vi "Formate into SQL Report.vi"(8 "error in (no error)":errorcluster) -> (0 "error out":errorcluster, 3 "Result for SQl Without Header":string[][](array[string]))   [LabVIEW 2017]
uses:
  <vilib>/Utility/file.llb/Read Delimited Spreadsheet (string).vi
panel:
  in  "file path (dialog if empty)":path=path "D:/STD EOL/MSSQL Report Viewer/IOT/Report/Sample Reports/Report/Test Report/Main Reports/21-05-19.csv"
  in  "Excepted Value":string="Excepted Value"
  in  "Test Type":string="Test type"
  out "Result wiht Header":string[][](array[string])
  in  "Variant":string="variant"
  in  "Model":string="Y1k"
  in  "Shift":string="A"
  in  "User Name":string="mmk"
  in  "Barcode":string="123"
  out "all rows":string[][](array[string])
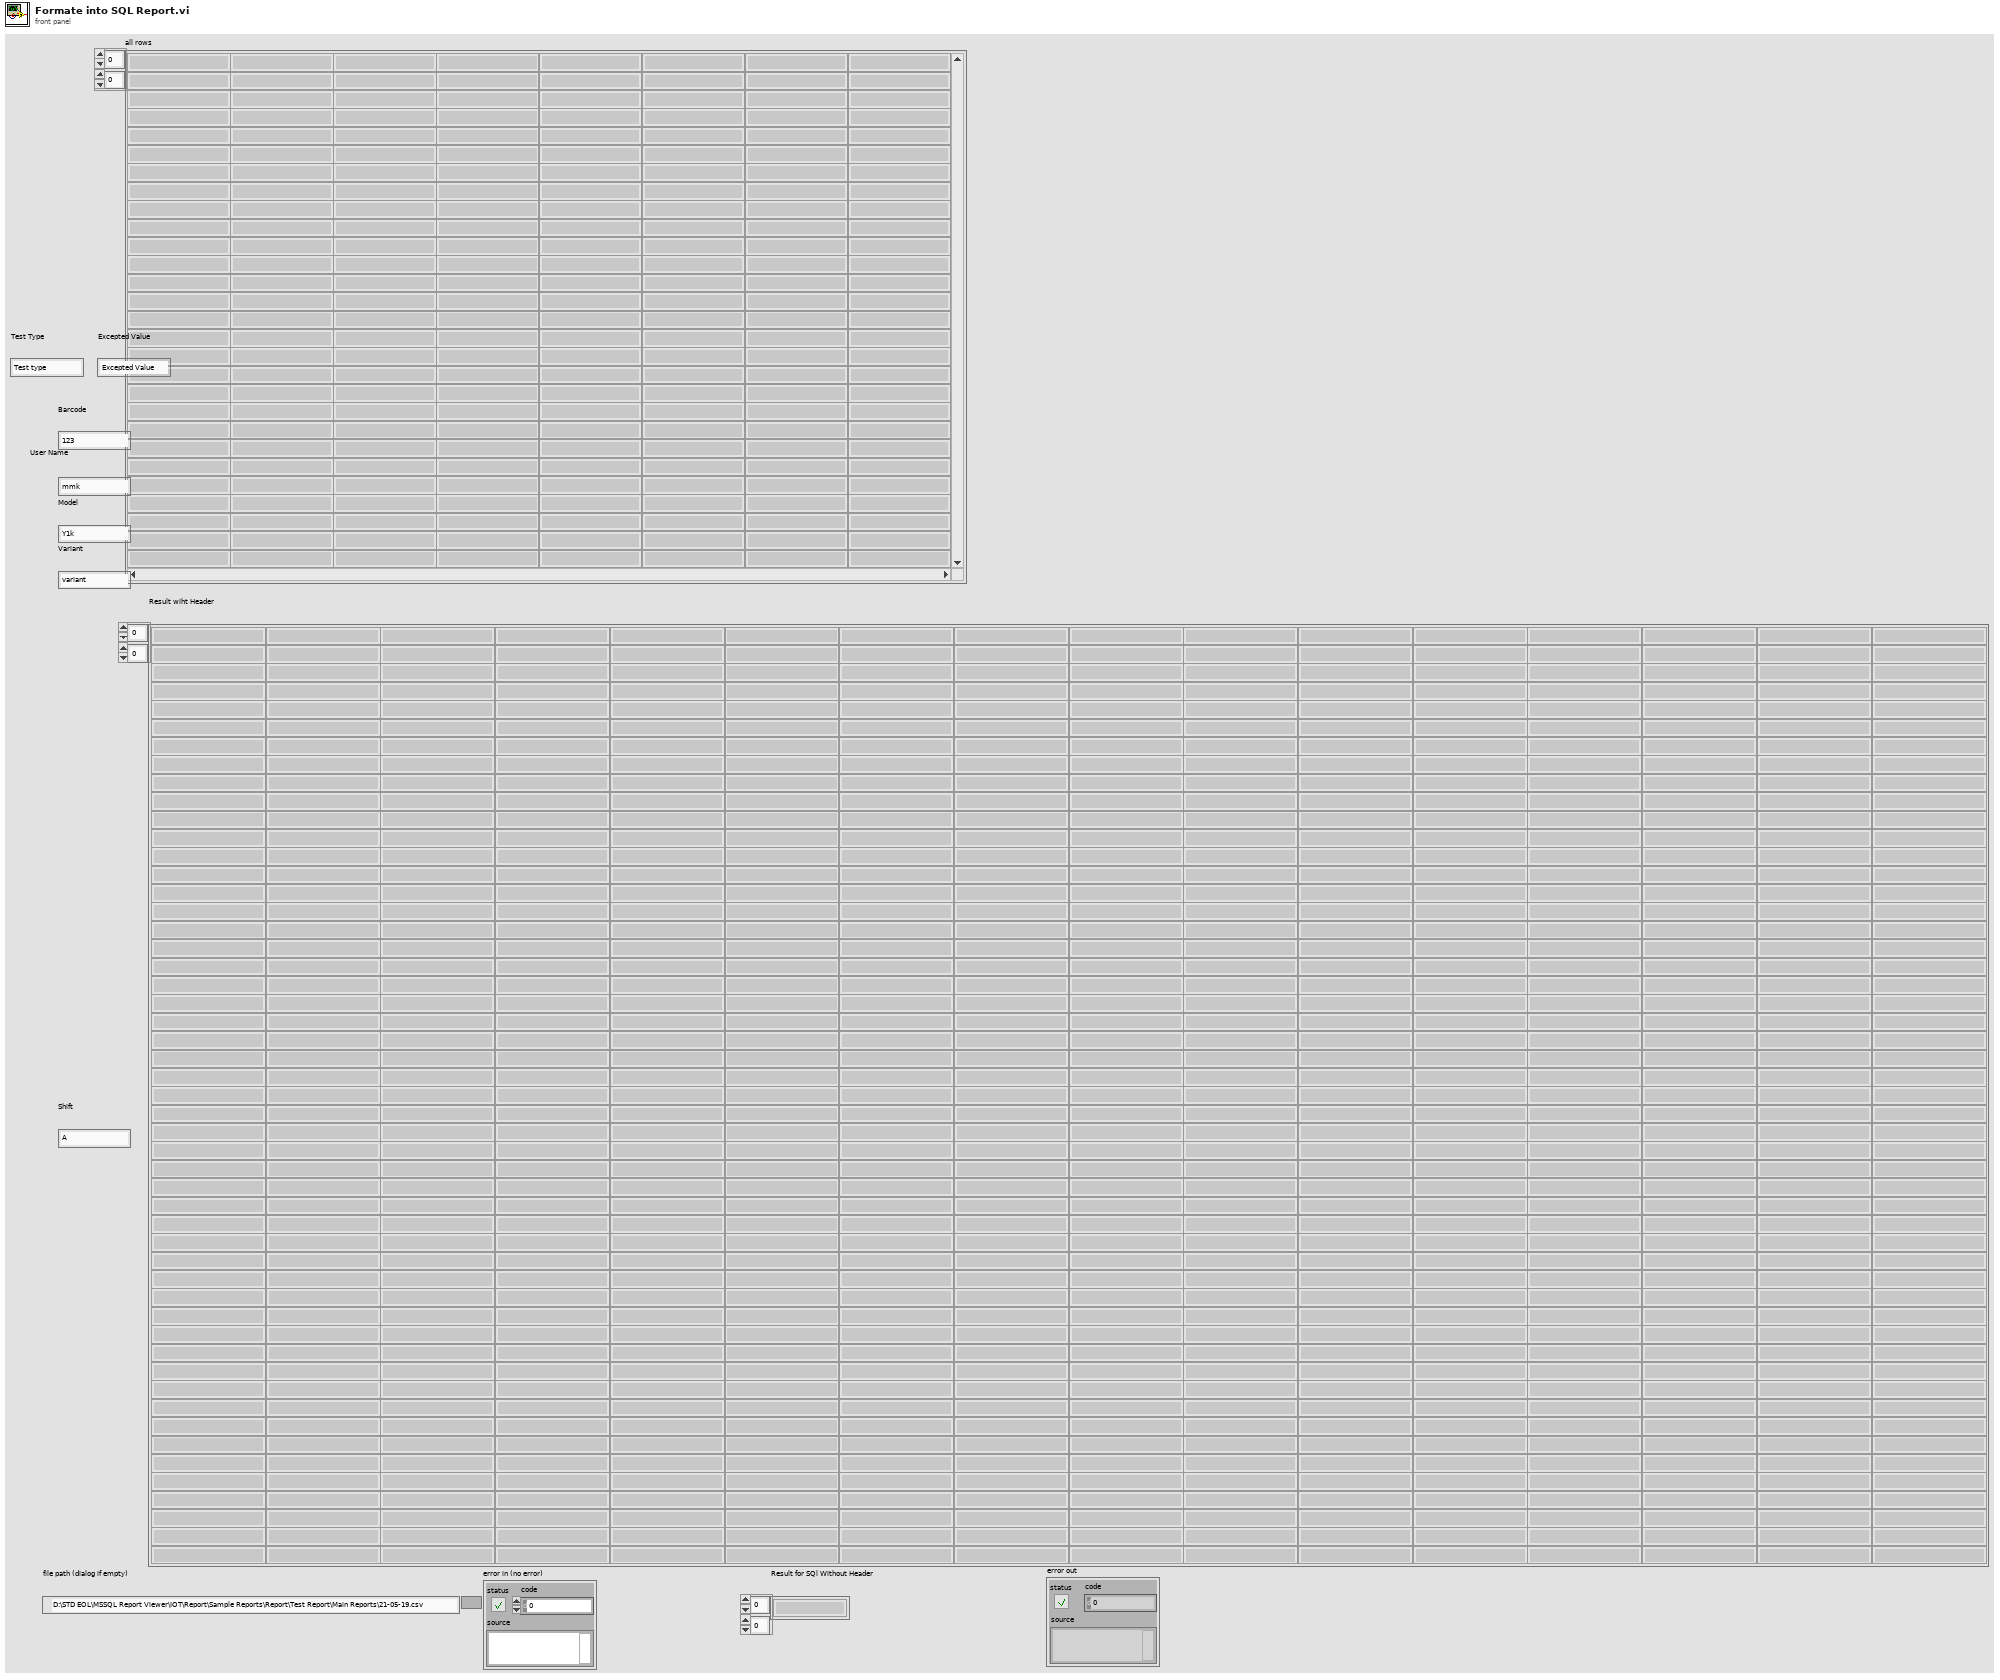
[diagram p1: front panel]
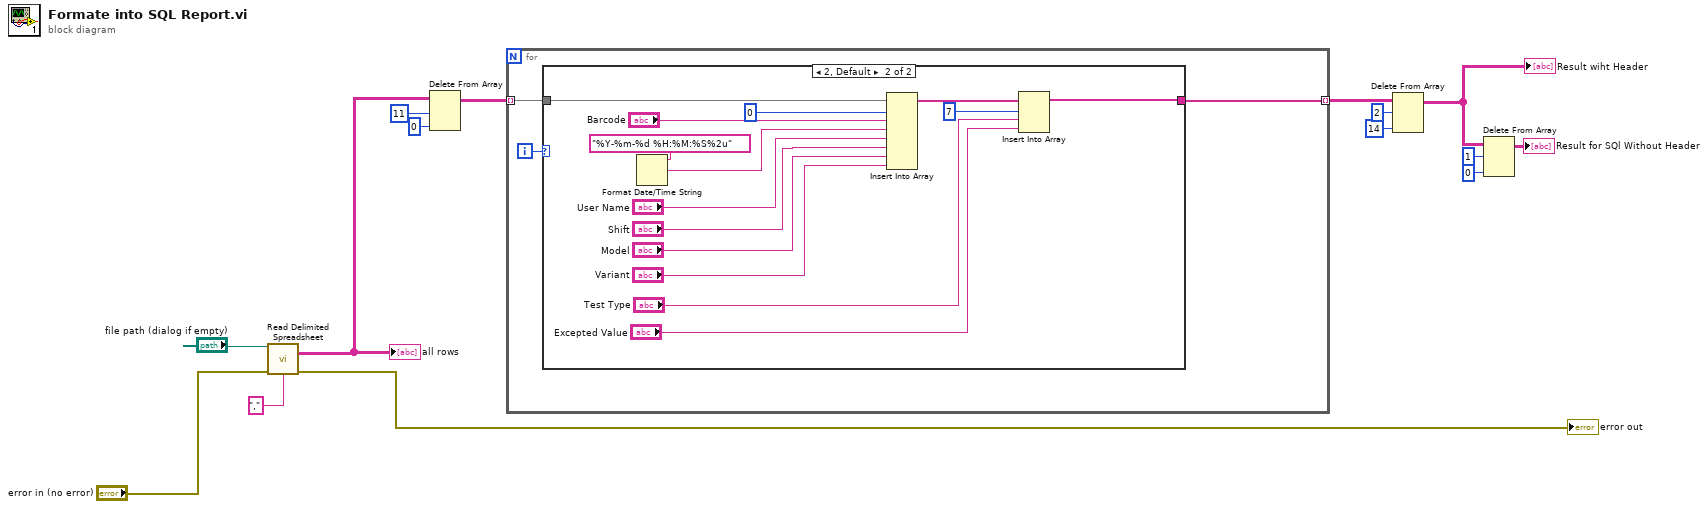
[diagram p0: block diagram]
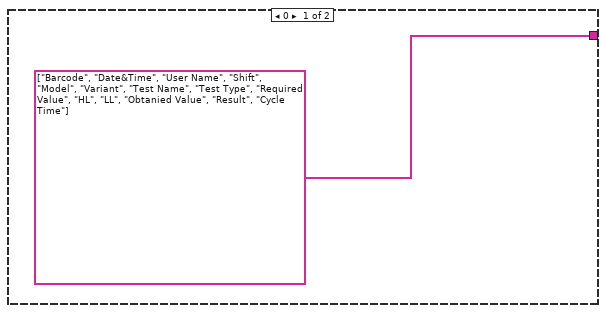
[diagram p2: hidden frame]
diagram:
  n1 = call-poly <vilib>:"Read Delimited Spreadsheet.vi"("file path (dialog if empty)"="file path (dialog if empty)", "error in (no error)"="error in (no error)", "delimiter (\\t)"="," ("delimiter (\\t)")) -> ("all rows"=w14:string[][], "error out"=→"error out":errorcluster)  [unwired: 7 in, 4 out]
  "all rows" <- w14
  n2 = Delete From Array(array=w14, length=11, index (col)=0 ("disabled index (col)")) -> (array with subset deleted=w13:string[][])  [unwired: 1 in, 1 out]
  n3 = for {
    tunnel: w13 -> [w18] mode=indexing
    tunnel: [w17] -> w10 mode=indexing
    i -> [w16]
    n4 = case shown="2, Default" w16 {
      tunnel: w18 -> [_ w33]
      tunnel: [string[] ["Barcode", "Date&Time", "User Name", "Shift", "Model", "Variant", "Test Name", "Test Type", "Required Value", "HL", "LL", "Obtanied Value", "Result", "Cycle Time"] w22] -> w17
      frame 0 {
      }
      frame 2, Default {
        n5 = Format Date/Time String(time format string (%c)="%Y-%m-%d %H:%M:%S%2u") -> (date/time string=w20:string)  [unwired: 2 in]
        n6 = Insert Into Array(array=w33, index=0, new element #1="Barcode", new element #2=w20, new element #3="User Name", new element #4="Shift", new element #5="Model", new element #6="Variant") -> (w26:string[])
        n7 = Insert Into Array(array=w26, index=7, new element #1="Test Type", new element #2="Excepted Value") -> (w22:string[])
      }
    }
  }
  n8 = Delete From Array(array=w10, length=2, index (col)=14 ("disabled index (col)")) -> (array with subset deleted=w7:string[][])  [unwired: 1 in, 1 out]
  "Result wiht Header" <- w7
  n9 = Delete From Array(array=w7, length=1, index (col)=0 ("disabled index (col)")) -> (array with subset deleted=→"Result for SQl Without Header":string[][])  [unwired: 1 in, 1 out]
